vi "GA_Crossover.vi"(6 "Parameters":T1={"Population size"=100, "Generations no."=500, "Significant digits"=4, "Crossover probabality"=0.85, "Mutation mode"=enum."one-point, fixed rate", "Use Gray code?"=FALSE, "Mutation rate"=0.05, "Min mutation rate"=0.0005, "Max mutation rate"=0.25, "Reproduction plan"=enum."Steady-state-replace-worst", "Elitism"=FALSE, "Fmax"=1} {"Max mutation rate" min=0.0 max=1.0; "Min mutation rate" min=0.0 max=1.0; "Mutation rate" min=0.0 max=1.0; "Crossover probabality" min=0.0 max=1.0; "Significant digits" min=1; "Generations no." min=1; "Population size" min=1}, 10 "Genotype 2":i8[](array[numeric]), 11 "Genotype 1":i8[](array[numeric])) -> (2 "Offspring 2":i8[](array[numeric]), 3 "Offspring 1":i8[](array[numeric]))   [LabVIEW 2016, in "Optimal Frequency Bands Search.lvlib" / "GeneticAlgorithm.lvlib"]
doc: "Процедура обмена генами в процессе скрещивания (кроссовера)"
uses:
  GeneticAlgorithm.lvlib
  GA_tParameters.ctl
panel:
  # "This VI is a part of BCI Design library, http://www.ru-bci.org \nCopyright © 2020, Sotnikov Peter, All rights reserved. License: CC BY-NC 4.0"
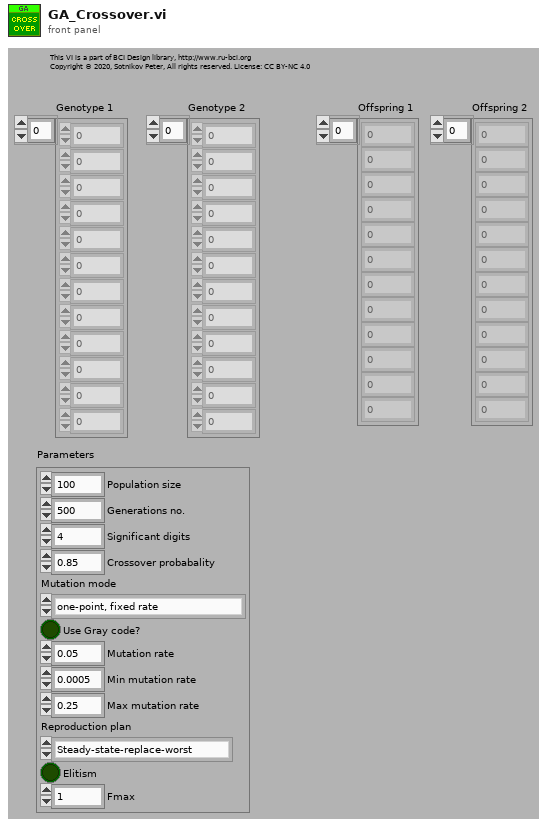
[diagram p1: front panel]
types:
  T1 = typedef "Optimal Frequency Bands Search.lvlib/GeneticAlgorithm.lvlib/GA_tParameters.ctl" = cluster{"Population size":i32, "Generations no.":i32, "Significant digits":i32, "Crossover probabality":dbl, "Mutation mode":enum16{"one-point, fixed rate", "one-point, fitness-adjustable rate", "one-point, distance-adjustable rate"}, "Use Gray code?":bool, "Mutation rate":dbl, "Min mutation rate":dbl, "Max mutation rate":dbl, "Reproduction plan":enum16{"Full generational replacement", "Steady-state-replace-random", "Steady-state-replace-worst"}, "Elitism":bool, "Fmax":i32}
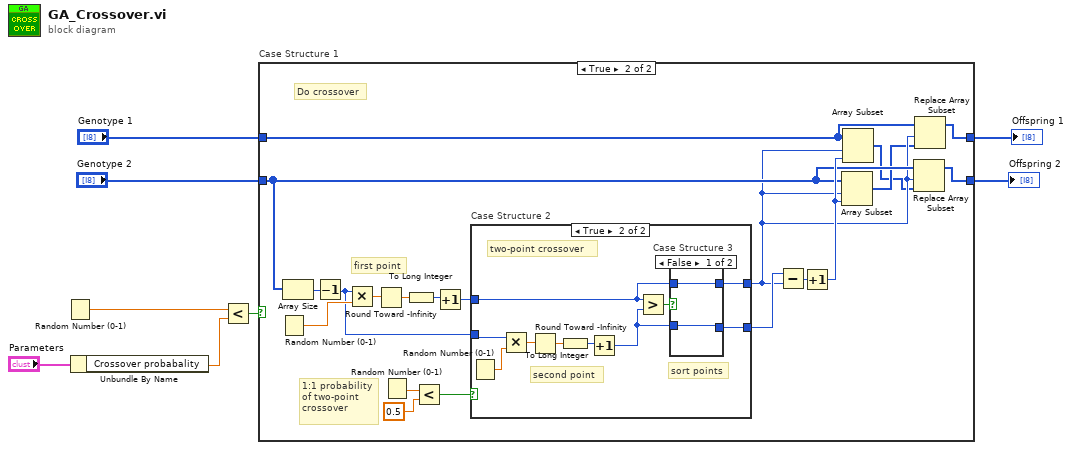
[diagram p0: block diagram]
diagram:
  n1 = Random Number (0-1)() -> (number: 0 to 1=w8:dbl)
  n2 = Unbundle By Name("Parameters") -> ("Crossover probabality"=w1:dbl)
  n3 = Less?(x=w8, y=w1) -> (x < y?=w7:bool)
  n4 = case "Case Structure 1" shown="True" w7 {
    tunnel: [w10 w13] -> w4
    tunnel: "Genotype 1" -> [w10 w17]
    tunnel: [w9 w14] -> w3
    tunnel: "Genotype 2" -> [w9 w16]
    frame False {
      # "no crossover"
    }
    frame True {
      # "1:1 probability\nof two-point\ncrossover"
      # "Do crossover"
      # "first point"
      n5 = Random Number (0-1)() -> (number: 0 to 1=w26:dbl)
      n6 = Array Size(array=w16) -> (size(s)=w27:i32)
      n7 = Decrement(x=w27) -> (x-1=w21:i32)
      n8 = Multiply(x=w21, y=w26) -> (x*y=w25:dbl)
      n9 = Round Toward -Infinity(1:w25) -> (0:w24:dbl)
      n10 = Random Number (0-1)() -> (number: 0 to 1=w30:dbl)
      n11 = To Long Integer(number=w24) -> (32bit integer=w23:i32)
      n12 = Less?(x=w30, y=0.5) -> (x < y?=w28:bool)
      n13 = Increment(x=w23) -> (x+1=w22:i32)
      n14 = case "Case Structure 2" shown="True" w28 {
        tunnel: w22 -> [w32 w36]
        tunnel: w21 -> [w31 w39]
        tunnel: [w32 w34] -> w15
        tunnel: [w31 w33] -> w20
        frame False {
          # "one-point crossover"
        }
        frame True {
          # "sort points"
          # "two-point crossover"
          # "second point"
          n15 = Random Number (0-1)() -> (number: 0 to 1=w38:dbl)
          n16 = Multiply(x=w39, y=w38) -> (x*y=w40:dbl)
          n17 = Round Toward -Infinity(1:w40) -> (0:w41:dbl)
          n18 = To Long Integer(number=w41) -> (32bit integer=w42:i32)
          n19 = Increment(x=w42) -> (x+1=w35:i32)
          n20 = Greater?(x=w36, y=w35) -> (0:w37:bool)
          n21 = case "Case Structure 3" shown="False" w37 {
            tunnel: w36 -> [w44 w46]
            tunnel: w35 -> [w43 w45]
            tunnel: [w43 w46] -> w33
            tunnel: [w44 w45] -> w34
            frame False {
            }
            frame True {
            }
          }
        }
      }
      n22 = Subtract(x=w20, y=w15) -> (x-y=w19:i32)
      n23 = Increment(x=w19) -> (x+1=w18:i32)
      n24 = Array Subset(array=w16, index=w15, length=w18) -> (w12:i8[])
      n25 = Array Subset(array=w17, index=w15, length=w18) -> (w11:i8[])
      n26 = Replace Array Subset(array=w16, new element=w11, index=w15) -> (w14:i8[])
      n27 = Replace Array Subset(array=w17, new element=w12, index=w15) -> (w13:i8[])
    }
  }
  "Offspring 1" <- w4
  "Offspring 2" <- w3
